vi "LoggingWindow.vi"() -> ()   [LabVIEW 2016]
uses:
  <vilib>/drjdpowell/SQLite Library/SQL Connection/Open (path).vi
  <vilib>/drjdpowell/SQLite Library/SQL Connection/Open (string).vi
  <vilib>/AdvancedString/Path To Command Line String.vi
  <vilib>/drjdpowell/SQLite Library/SQL Connection/Connection.lvclass
  <vilib>/NI/Progress Bar/Progress Bar.lvlib
panel:
  in  "Tab Control":enum32{"Page 1", "Page 2"}(tab)
  in  "Enter":bool
  in  "User Name":string
  in  "Password":string
  in  "Login":bool
  in  "Reset":bool
  in  "Close":bool
  out "error out":errorcluster
  # "WELCOME TO THE WORLD OF AUTOMATION"
  # "Please Enter your Username & Password"
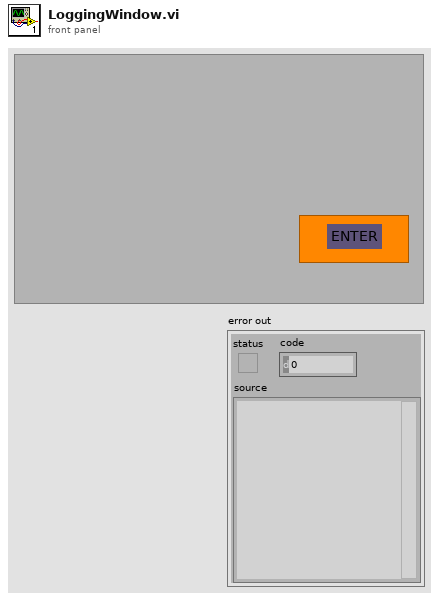
[diagram p1: front panel]
types:
  T1 = cluster{"Result Set[0]":string, "Result Set[1]":string, "Result Set[2]":string, "Result Set[3]":string, "Result Set[4]":string, "Result Set[5]":string, "Result Set[6]":string, "Result Set[7]":string, "Result Set[8]":string}
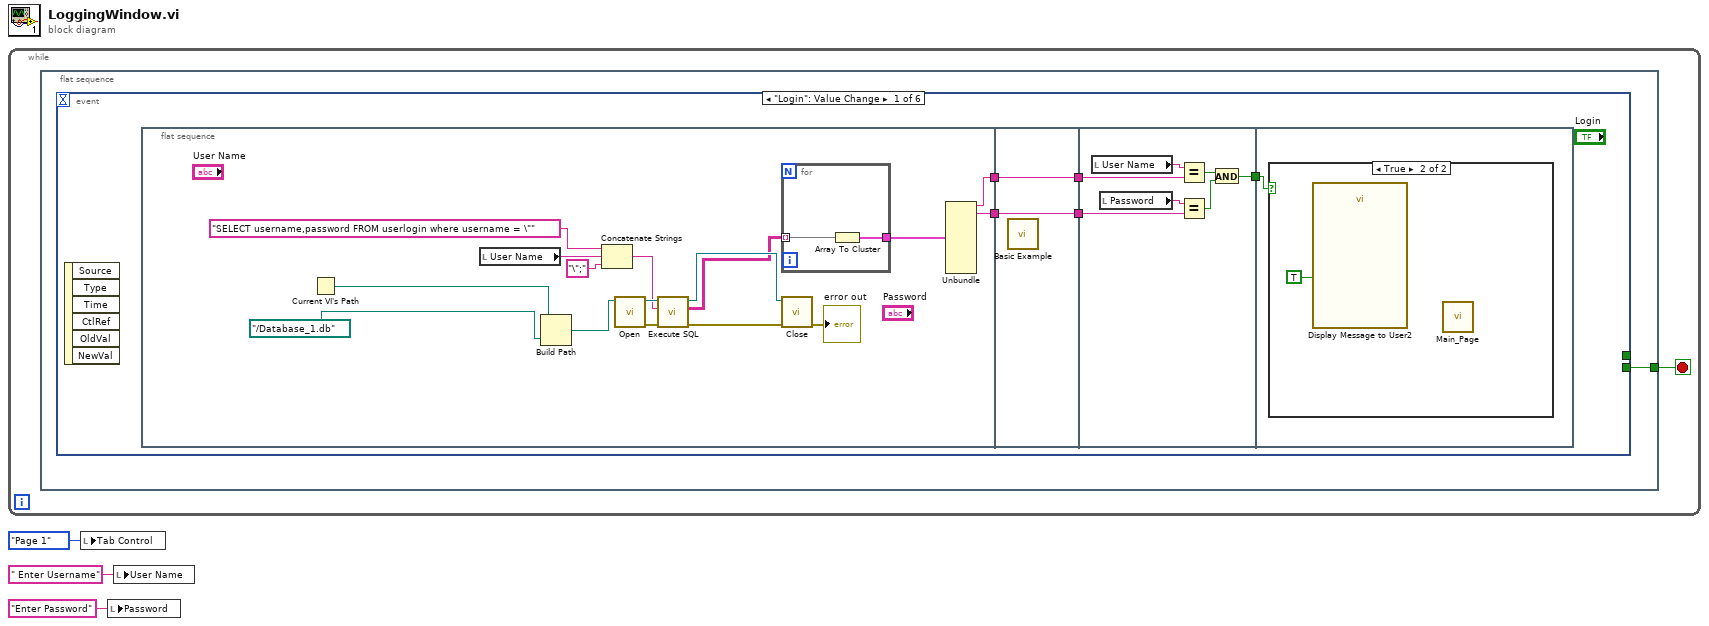
[diagram p0: block diagram]
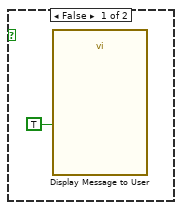
[diagram p2: hidden frame]
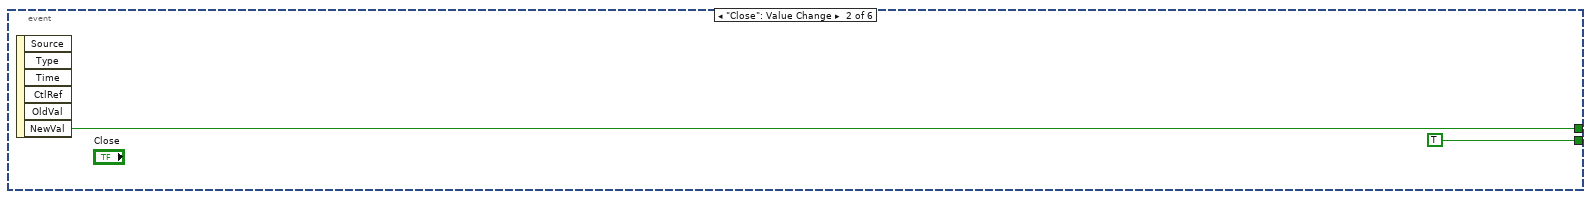
[diagram p3: hidden frame]
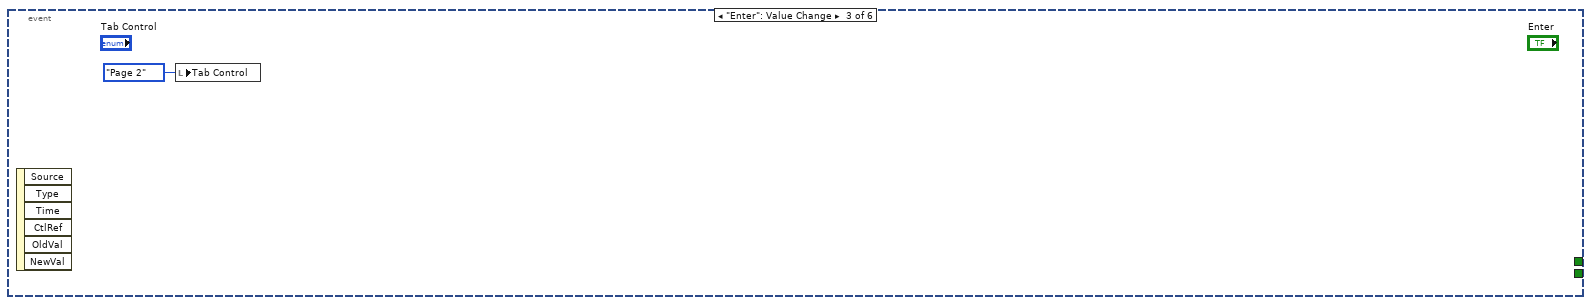
[diagram p4: hidden frame]
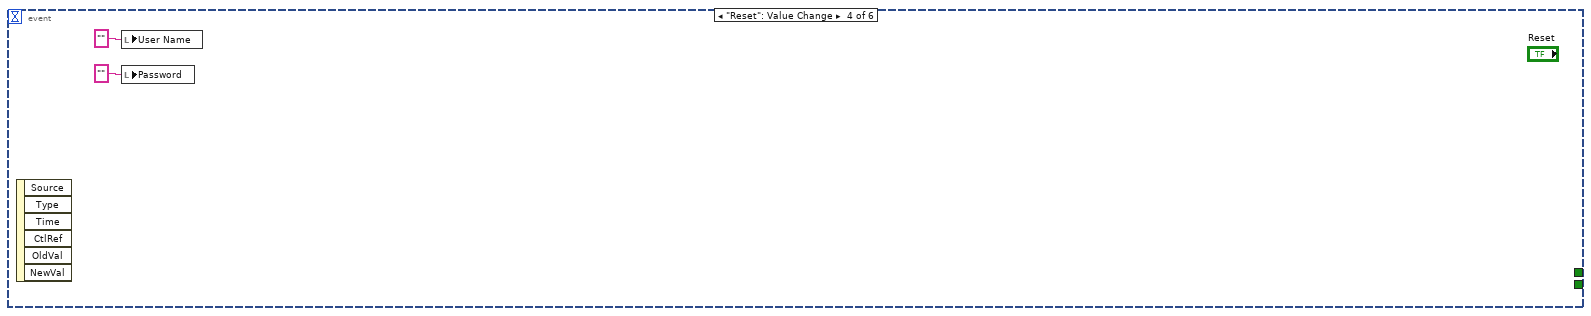
[diagram p5: hidden frame]
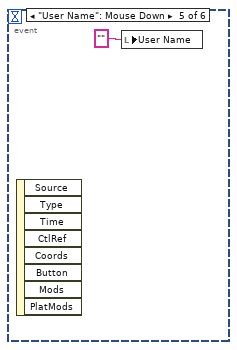
[diagram p6: hidden frame]
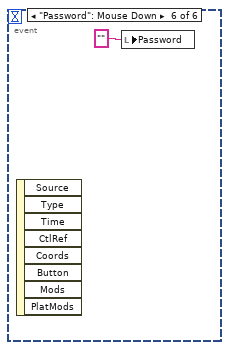
[diagram p7: hidden frame]
diagram:
  n1 = while {
    stop <- w4 stop-if-true
    n2 = flat-sequence {
      tunnel: [w5] -> w4
      frame #0 {
        n3 = event shown="[0] \"Login\": Value Change" {
          selector: _ -> [_ _ _ _ _ _]
          dyn-events: _ -> [_ _ _ _ _ _]
          timeout: _ -> [_ _ _ _ _ _]
          tunnel: [_ TRUE _ _ _ _] -> w5
          tunnel: [_ w41 _ _ _ _] -> _
          event "Login": Value Change {
            n4 = event-data() -> ()  [unwired: 1 in, 6 out]
            n5 = flat-sequence {
              tunnel: [w15] -> w8
              tunnel: [w14] -> w6
              tunnel: [w30] -> w9
              tunnel: w8 -> [w30]
              tunnel: [w29] -> w7
              tunnel: w6 -> [w29]
              tunnel: [w35] -> w10
              tunnel: w9 -> [w32]
              tunnel: w7 -> [w31]
              tunnel: w10 -> [w38]
              frame #0 {
                n6 = Current VI's Path() -> (path=w11:path)
                n7 = local read "User Name"() -> (w19:string)
                n8 = Build Path(base path=w11, name or relative path=path "../Database_1.db") -> (appended path=w13:path)
                n9 = Concatenate Strings("SELECT username,password FROM userlogin where username = \"", w19, "\";") -> (w21:string)
                n10 = call-poly <vilib>:"Open.vi"("db file"=w13) -> ("error out"=w23:errorcluster, "SQLite Connection"=w24:refnum<class "Connection.lvclass">)  [unwired: 9 in]
                n11 = call <vilib>:"Execute SQL.vi"("error in (no error)"=w23, "SQL"=w21, "SQLite Connection in"=w24) -> ("error out"=w25:errorcluster, "Result Set"=w16:string[][], "SQLite Connection"=w26:refnum<class "Connection.lvclass">)  [unwired: 5 in, 1 out]
                n12 = for {
                  tunnel: [w28] -> w17
                  tunnel: w16 -> [w27] mode=indexing
                  n13 = Array To Cluster(array=w27) -> (cluster=w28:T1)
                }
                n14 = call-dynamic "Close.vi"("error in (no error)"=w25, "SQLite Connection in"=w26) -> ("error out"=→"error out":errorcluster)  [unwired: 9 in]
                n15 = Unbundle(w17) -> ("Result Set[0]"=w14:string, "Result Set[1]"=w15:string)  [unwired: 7 out]
              }
              frame #1 {
                n16 = call <vilib>:"Basic Example.vi"() -> ()  [unwired: 12 in]
              }
              frame #2 {
                n17 = local read "User Name"() -> (w34:string)
                n18 = local read "Password"() -> (w33:string)
                n19 = Equal?(x=w34, y=w31) -> (x = y?=w36:bool)
                n20 = Equal?(x=w33, y=w32) -> (x = y?=w37:bool)
                n21 = And(x=w36, y=w37) -> (x .and. y?=w35:bool)
              }
              frame #3 {
                n22 = case shown="True" w38 {
                  frame False {
                    n23 = call "Display Message to User"("Enable"=TRUE) -> ()  [unwired: 9 in, 2 out]
                  }
                  frame True {
                    n24 = call "Display Message to User2"("Enable"=TRUE) -> ()  [unwired: 9 in, 2 out]
                    n25 = call "Main_Page.vi"() -> ()  [unwired: 12 in]
                  }
                }
              }
            }
          }
          event "Close": Value Change {
            n26 = event-data() -> ("NewVal"=w41:bool)  [unwired: 1 in, 5 out]
          }
          event "Enter": Value Change {
            n27 = event-data() -> ()  [unwired: 1 in, 6 out]
            n28 = local write "Tab Control"(enum32{"Page 1", "Page 2"}."Page 2" ("Tab Control")) -> ()
          }
          event "Reset": Value Change {
            n29 = event-data() -> ()  [unwired: 1 in, 6 out]
            n30 = local write "User Name"("" ("User Name")) -> ()
            n31 = local write "Password"("" ("Password")) -> ()
          }
          event "User Name": Mouse Down {
            n32 = event-data() -> ()  [unwired: 1 in, 8 out]
            n33 = local write "User Name"("" ("User Name")) -> ()
          }
          event "Password": Mouse Down {
            n34 = event-data() -> ()  [unwired: 1 in, 8 out]
            n35 = local write "Password"("" ("Password")) -> ()
          }
        }
      }
    }
  }
  n36 = local write "Tab Control"(enum32{"Page 1", "Page 2"}."Page 1" ("Tab Control")) -> ()
  n37 = local write "Password"("Enter Password" ("Password")) -> ()
  n38 = local write "User Name"(" Enter Username" ("User Name")) -> ()
